vi "User Access Level FGV.vi"(7 "User Level Cmd":T1, 8 "Error In":errorcluster, 10 "User Name":string) -> (0 "Error Out":errorcluster, 1 "User Level":string)   [LabVIEW 2017]
doc: "This FGV holds the Access Level for the user currently logged in. It executes the following methods:\n\n1. <B>Read User Access Level File:</B> Reads a tab-delimited text file containing User Names and corresponding Access Levels.\n2. <B>Set Current Access Level:</B> Sets the Access level for the User Name input.\n3. <B>Get Current Access Level:</B> Returns the Access level for the current User."
uses:
  User Level Cmd.ctl
  <vilib>/Utility/file.llb/Read Delimited Spreadsheet (string).vi
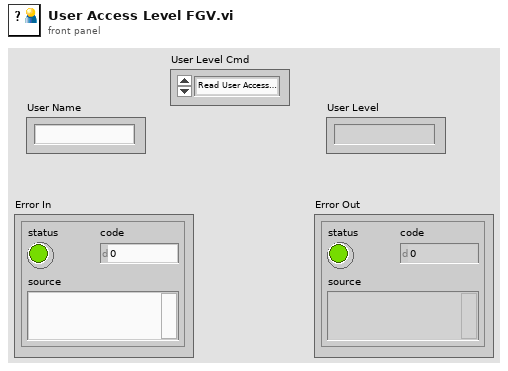
[diagram p1: front panel]
types:
  T1 = typedef "User Level Cmd.ctl" = enum16{"Read User Access Level File", "Set Current User", "Get User Access Level"}
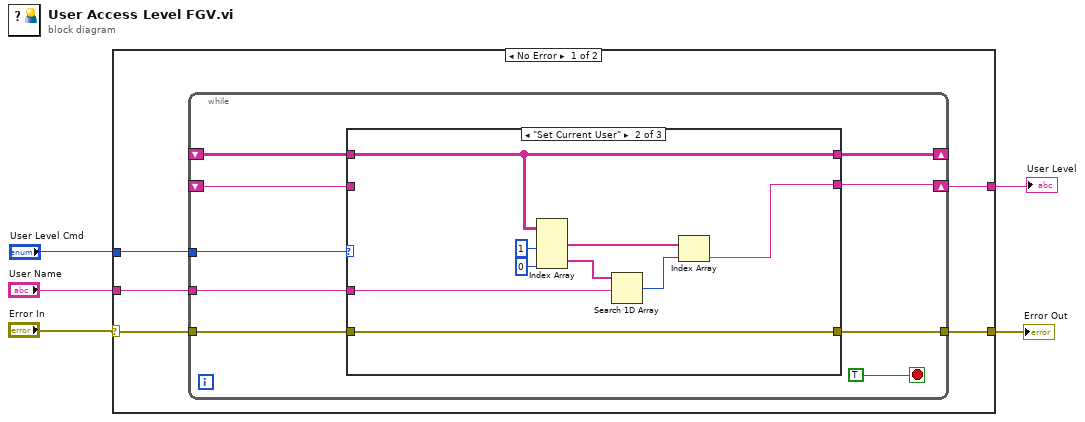
[diagram p0: block diagram]
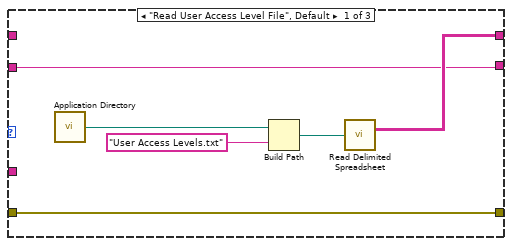
[diagram p2: hidden frame]
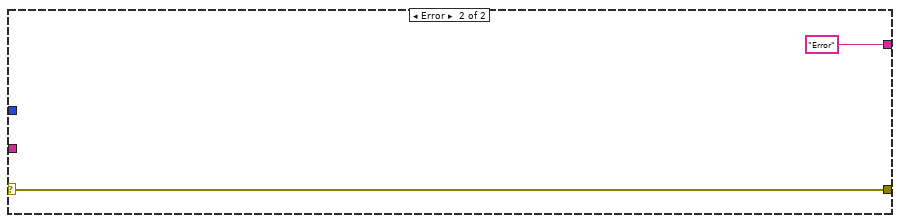
[diagram p4: hidden frame]
diagram:
  n1 = case shown="No Error" "Error In" {
    selector: "Error In" -> [w9 w39]
    tunnel: "User Level Cmd" -> [w10 _]
    tunnel: "User Name" -> [w8 _]
    tunnel: [w7 "Error"] -> w2
    tunnel: [w6 w39] -> w1
    frame No Error {
      n2 = while {
        tunnel: w10 -> [w18]
        tunnel: w9 -> [w17]
        tunnel: [w16] -> w6
        shift-right: [w14] -> _
        shift-left: _ -> [w15]
        tunnel: w8 -> [w13]
        shift-right: [w12] -> w7
        shift-left: _ -> [w11]
        stop <- TRUE ("Stop Button") stop-if-true
        n3 = case shown="\"Set Current User\"" w18 {
          tunnel: w17 -> [w25 w34 w37]
          tunnel: [w25 w34 w37] -> w16
          tunnel: w15 -> [_ w33 w36]
          tunnel: [w21 w33 w36] -> w14
          tunnel: w13 -> [_ w30 _]
          tunnel: [w20 w28 w35] -> w12
          tunnel: w11 -> [w20 _ w35]
          frame "Read User Access Level File", Default {
            n4 = call <vilib>:"Application Directory.vi"() -> ("Application Directory"=w23:path)
            n5 = Build Path(base path=w23, name or relative path="User Access Levels.txt") -> (appended path=w22:path)
            n6 = call-poly <vilib>:"Read Delimited Spreadsheet.vi"("file path (dialog if empty)"=w22) -> ("all rows"=w21:string[][])  [unwired: 9 in, 5 out]
          }
          frame "Set Current User" {
            n7 = Index Array(array=w33, index (col) #1=1 ("disabled index (col)"), index (col) #2=0 ("index (col)")) -> (element #1=w31:string[], element #2=w32:string[])  [unwired: 2 in]
            n8 = Search 1D Array(1D array=w32, element=w30) -> (index of element=w29:i32)  [unwired: 1 in]
            n9 = Index Array(array=w31, index=w29) -> (element=w28:string)
          }
          frame "Get User Access Level" {
          }
        }
      }
    }
    frame Error {
    }
  }
  "User Level" <- w2
  "Error Out" <- w1
